vi "Apply Web Service Settings.vi"(8 "error in (no error)":errorcluster, 11 "LabVIEW Web Service Request":refnum<class "Web Request.lvclass">) -> (0 "error out":errorcluster, 3 "LabVIEW Web Service Request out":refnum<class "Web Request.lvclass">)   [LabVIEW 2023]
doc: "Applies the settings currently configured in the <B>Web Service Settings Store.vi</B> to a web service response."
uses:
  <vilib>/wsapi/Web Request.lvclass
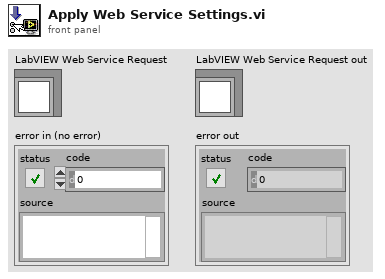
[diagram p1: front panel]
types:
  T1 = typedef "Web Service Settings.ctl" = cluster{"Enable CORS":bool}
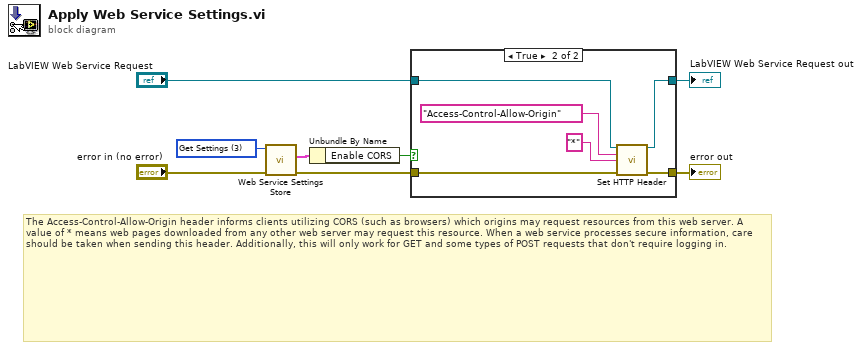
[diagram p0: block diagram]
diagram:
  w8 = u16 3 items=["Initialize Settings Store", "Destroy Settings Store", "Set Settings", "Get Settings"] ("action")
  # "The Access-Control-Allow-Origin header informs clients utilizing CORS (such as browsers) which origins may request resources from this web server. A value of * means web pages downloaded from any other web server may request this resource. When a web service processes secure information, care should be taken when sending this header. Additionally, this will only work for GET and some types of POST requests that don't require logging in."
  n1 = call "Web Service Settings Store.vi"("error in (no error)"="error in (no error)", "action"=w8) -> ("error out"=w6:errorcluster, "settings out"=w5:T1)  [unwired: 8 in]
  n2 = Unbundle By Name(w5) -> ("Enable CORS"=w1:bool)
  n3 = case shown="True" w1 {
    tunnel: w6 -> [w10 w16]
    tunnel: [w10 w15] -> w4
    tunnel: "LabVIEW Web Service Request" -> [w9 w14]
    tunnel: [w9 w13] -> w2
    frame False {
    }
    frame True {
      n4 = call <vilib>:"Set HTTP Header.vi"("LabVIEW Web Service Request"=w14, "header"="Access-Control-Allow-Origin", "header value"="*", "error in (no error)"=w16) -> ("LabVIEW Web Service Request out"=w13:refnum<class "Web Request.lvclass">, "error out"=w15:errorcluster)  [unwired: 10 in]
    }
  }
  "error out" <- w4
  "LabVIEW Web Service Request out" <- w2
